vi "Fetch Voltage.vi"(0 "VISA resource name":refnum<visa-resource-name>, 11 "error in (no error)":errorcluster) -> (2 "Average Voltage":dbl, 3 "RMS Voltage":dbl, 4 "VISA resource name out":refnum<visa-resource-name>, 6 "High Voltage Level":dbl, 8 "Low Voltage Level":dbl, 13 "Maximum Voltage Level":dbl, 14 "Minimum Voltage Level":dbl, 15 "error out":errorcluster)   [LabVIEW 2019, in "Agilent N7976A.lvlib"]
doc: "Fetches voltage information from the instrument.\n\nNote:\nUse this VI only with other low-level VIs. The high-level VIs automatically incorporate this functionality. This VI does not check the instrument status."
uses:
  <instrlib>/Agilent N7976A/Agilent N7976A.lvlib
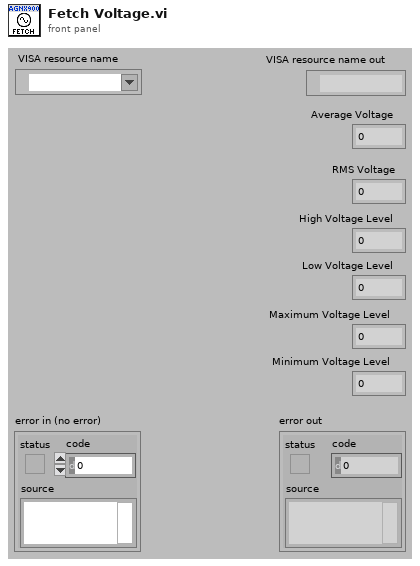
[diagram p1: front panel]
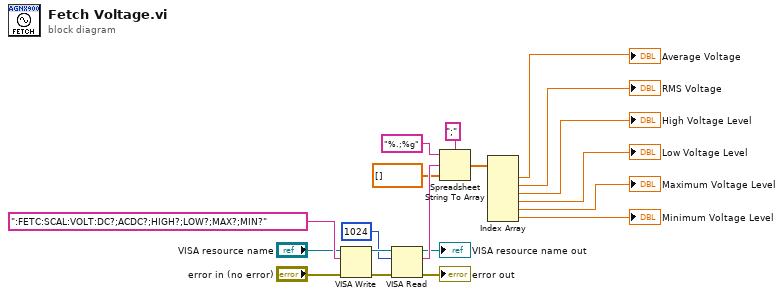
[diagram p0: block diagram]
diagram:
  n1 = VISA Write(VISA resource name="VISA resource name", write buffer=":FETC:SCAL:VOLT:DC?;ACDC?;HIGH?;LOW?;MAX?;MIN?", error in (no error)="error in (no error)") -> (VISA resource name out=w18:refnum<visa-resource-name>, error out=w19:errorcluster)  [unwired: 1 out]
  n2 = VISA Read(VISA resource name=w18, byte count=u32 1024, error in (no error)=w19) -> (VISA resource name out=→"VISA resource name out":refnum<visa-resource-name>, read buffer=w16:string, error out=→"error out":errorcluster)  [unwired: 1 out]
  n3 = Spreadsheet String To Array(delimiter (Tab)=";", format string="%.;%g", spreadsheet string=w16, array type (2D Dbl)=dbl[] []) -> (array=w13:dbl[])
  n4 = Index Array(array=w13) -> (element #1=→"Average Voltage":dbl, element #2=→"RMS Voltage":dbl, element #3=→"High Voltage Level":dbl, element #4=→"Low Voltage Level":dbl, element #5=→"Maximum Voltage Level":dbl, element #6=→"Minimum Voltage Level":dbl)  [unwired: 6 in]
